vi "EventDetectionMode plane.vi"(8 "error in (no error)":errorcluster, 11 "SetupInfo_IN":T1={"ConfigParameters_Analog"={"JAI camera fps"=240.0, "Bi-Lateral Galvo xy scan range (V)"=0.7, "Bi-Lateral Galvo xy scan frequency (Hz)"=500, "AOM Blind percent (%)"=0.1, "AOM start blind percent (%) "=70.0, "ROI threshold"=1.0, "AO Sampling rate"=1000000.0}, "ConfigParameters_Digital"={"Steps per volume"=25.0, "Time per volume (s)"=0.4, "OG start layer"=15.0, "Objective Lin Rising Vel (micron/ms）"=1.0, "Image depth (micron)"=200.0, "OG latency (s)"=10.0, "OG repitation"=3.0, "OG end layer"=17.0, "Shock1 duration (s)"=0.001, "Shock2 duration (s)"=0.001, "Shock3 duration (s)"=0.01, "Shock4 duration (s)"=0.01, "Shock5 duration (s)"=0.1, "Shock duration_New"=[]}, "ConfigParameters_Other1"={"Frontal Galvo xy scan range (V)"=0.14, "Frontal Galvo xy scan frequency (Hz)"=500, "PFI 0 digital clock frequency"=500000.0, "Window size for layer index"=0.5, "sCMOS fps"=95.0}, "ConfigParameters_Others2"={"#Trials baseline"=6, "#Trials test"=6, "Time before acq. (s)"=360.0, "Time before test (s)"=600.0, "#Blocks acquisition"=5, "Inter-trial interval baseline (s)"=60.0, "#Trials per acquition block"=6, "Inter-block interval acquisition (s)"=360.0, "Inter-trial interval acquisition (s)"=20.0, "Flash latency (s)"=10.0, "Flash duration (s)"=3.2, "Response duration (s)"=10.0, "MaxTimeEventDetection (s)"=6, "StimType"=enum."Flash", "#MaxEvents"=6}, "ProcessParametersOut"={"stand Z vol Acquisition time (s)"=0.2631578947368421, "stand Z vol Backward time (s)"=0.13684210526315793, "Objective scan volt"=5.0, "Bi-lateral Galvo Z scan volt"=0.1800000180000018, "Frontal Galvo Z scan volt"=0.14940000509752818, "Objective step length (micron)"=8.0, "OG Z volet Linear Dec time (s)"=0.024, "OG Z vol Stim. steps time (s)"=0.031578947368421054, "OG Z vol Linear Acc time (s)"=0.112, "#Vol. of flash"=8, "#Vol. of shock"=1, "#Vol. bef flash"=25, "#Vol. aft flash"=17, "OG Z vol Linear Dec time (s)"=0.112, "OG Z vol time (s)"=0.39073684210526316, "Stack duration"=[0.001, 0.001, 0.01, 0.01, 0.1], "AOM stand. value size"=400000, "Plane indexing length"=0, "#Vol. blank"=0, "#Vol. blank before acq"=1000000, "#Vol. blank before test"=263158, " #Inter-block interval acquisition (Ed-St Vol)"=1000000}, "WaveformParameters"={"stand Z vol Acquisition samp info"={"Fs"=1000000.0, "#s"=263158.0}, "stand Z vol Backward samp info"={"Fs"=1000000.0, "#s"=136842.0}, "OG Z vol Linear Acc samp info"={"Fs"=1000000.0, "#s"=112000.0}, "OG Z vol Stim. steps samp info"={"Fs"=1000000.0, "#s"=31579.0}, "OG Z volet Linear Dec samp info"={"Fs"=1000000.0, "#s"=24000.0}, "OG Z vol Linear Dec samp info"={"Fs"=1000000.0, "#s"=112000.0}, "OG Z vol samp info"={"Fs"=1000000.0, "#s"=390737.0}, "stand Z vol backforth samp info"={"Fs"=1000000.0, "#s"=400000.0}}, "AnalogWaveform"={"Bi-lateral Galvo Z stand waveform"={"t0"=timestamp(0 s since 1904-01-01), "dt"=1.0, "Y"=[]}, "Frontal Galvo Z stand waveform"={"t0"=timestamp(0 s since 1904-01-01), "dt"=1.0, "Y"=[]}, "Bi-lateral Galvo XY stand waveform"={"t0"=timestamp(0 s since 1904-01-01), "dt"=1.0, "Y"=[]}, "Frontal Galvo XY stand waveform"={"t0"=timestamp(0 s since 1904-01-01), "dt"=1.0, "Y"=[]}, "sCMOS stand waveform"={"t0"=timestamp(0 s since 1904-01-01), "dt"=1.0, "Y"=[]}, "Detection objective stand waveform"={"t0"=timestamp(0 s since 1904-01-01), "dt"=1.0, "Y"=[]}, "AOM stand waveform"={"t0"=timestamp(0 s since 1904-01-01), "dt"=1.0, "Y"=[]}, "PFI 0 clock stand waveform"={"t0"=timestamp(0 s since 1904-01-01), "dt"=1.0, "Y"=[]}, "Bi-lateral Galvo Z OG waveform"={"t0"=timestamp(0 s since 1904-01-01), "dt"=1.0, "Y"=[]}, "Bi-lateral Galvo XY OG waveform"={"t0"=timestamp(0 s since 1904-01-01), "dt"=1.0, "Y"=[]}, "Frontal Galvo Z OG waveform"={"t0"=timestamp(0 s since 1904-01-01), "dt"=1.0, "Y"=[]}, "Frontal Galvo XY OG waveform"={"t0"=timestamp(0 s since 1904-01-01), "dt"=1.0, "Y"=[]}, "sCMOS OG waveform"={"t0"=timestamp(0 s since 1904-01-01), "dt"=1.0, "Y"=[]}, "Detection objective OG waveform"={"t0"=timestamp(0 s since 1904-01-01), "dt"=1.0, "Y"=[]}, "AOM OG waveform"={"t0"=timestamp(0 s since 1904-01-01), "dt"=1.0, "Y"=[]}, "PFI 0 clock OG wavee"={"t0"=timestamp(0 s since 1904-01-01), "dt"=1.0, "Y"=[]}, "sCMOS blank waveform"={"t0"=timestamp(0 s since 1904-01-01), "dt"=1.0, "Y"=[]}, "All analog OG wave"=[], "All analog stand wave"=[], "All analog blank wave"=[], "BufferWaveform_Analog"=[], "Bi-lateral Galvo Z XY"={"t0"=timestamp(0 s since 1904-01-01), "dt"=1.0, "Y"=[]}, "Frontal Galvo Z XY"={"t0"=timestamp(0 s since 1904-01-01), "dt"=1.0, "Y"=[]}, "sCMOS Trigger XY"={"t0"=timestamp(0 s since 1904-01-01), "dt"=1.0, "Y"=[]}, "Detection objective XY"={"t0"=timestamp(0 s since 1904-01-01), "dt"=1.0, "Y"=[]}, "AOM XY"={"t0"=timestamp(0 s since 1904-01-01), "dt"=1.0, "Y"=[]}, "Analog_XY"=[]}, "DigitalWaveform"={"AllDigitalStandWave"=[], "AllDigialEvokedWave"=[], "AllDigialOGWave"=[], "AllDigitalPairWave_1"=[], "AllDigitalPairWave_2"=[], "AllDigitalPairWave_3"=[], "AllDigitalPairWave_4"=[], "AllDigitalPairWave_5"=[], "Plane Indexing"={"t0"=timestamp(0 s since 1904-01-01), "dt"=0.0, "Y"={"transitions"=[], "data"=[]}, "error"={"status"=FALSE, "code"=37421928, "source"=""}}, "Plane indexing P0.5 OG"={"t0"=timestamp(0 s since 1904-01-01), "dt"=0.0, "Y"={"transitions"=[], "data"=[]}, "error"={"status"=FALSE, "code"=37421928, "source"=""}}, "AllDigitalPairWaves"=[], "BufferWaveform_Digital"=[], "AllDigitalBlankWave"=[], "Digial_XY"=[], "Digital_XY_flash"=[], "Digial_XY DMD"=[]}, "PhysicalResource"={"PhysicalChannels_AI"="", "PhysicalChannels_AO"="", "PhysicalChannels_DO"="", "Task_AnalogOutput"="", "Task_DigitalOutput"="", "Task_AnalogInput"=""}, "ControlsRef"={"Mode_1"=refnum, "EventDetectionMode"=refnum, "Mode_2A"=refnum, "StimulationMode"=refnum, "Mode_2B"=refnum, "ErrorMeg"=refnum}, "test"=""} {"ConfigParameters_Other1"."Frontal Galvo xy scan frequency (Hz)" min=500 max=500; "ConfigParameters_Other1"."Frontal Galvo xy scan range (V)" min=0.0 max=1.5; "ConfigParameters_Analog"."AOM start blind percent (%)" min=10.0 max=90.0; "ConfigParameters_Analog"."AOM Blind percent (%)" min=0.1 max=100.0; "ConfigParameters_Analog"."Bi-Lateral Galvo xy scan frequency (Hz)" min=500 max=500; "ConfigParameters_Analog"."Bi-Lateral Galvo xy scan range (V)" min=0.0 max=1.5}) -> (0 "error out":errorcluster, 3 "SetupInfo_OUT":T1={"ConfigParameters_Analog"={"JAI camera fps"=240.0, "Bi-Lateral Galvo xy scan range (V)"=0.7, "Bi-Lateral Galvo xy scan frequency (Hz)"=500, "AOM Blind percent (%)"=0.1, "AOM start blind percent (%) "=70.0, "ROI threshold"=1.0, "AO Sampling rate"=1000000.0}, "ConfigParameters_Digital"={"Steps per volume"=25.0, "Time per volume (s)"=0.4, "OG start layer"=15.0, "Objective Lin Rising Vel (micron/ms）"=1.0, "Image depth (micron)"=200.0, "OG latency (s)"=10.0, "OG repitation"=3.0, "OG end layer"=17.0, "Shock1 duration (s)"=0.001, "Shock2 duration (s)"=0.001, "Shock3 duration (s)"=0.01, "Shock4 duration (s)"=0.01, "Shock5 duration (s)"=0.1, "Shock duration_New"=[]}, "ConfigParameters_Other1"={"Frontal Galvo xy scan range (V)"=0.14, "Frontal Galvo xy scan frequency (Hz)"=500, "PFI 0 digital clock frequency"=500000.0, "Window size for layer index"=0.5, "sCMOS fps"=95.0}, "ConfigParameters_Others2"={"#Trials baseline"=6, "#Trials test"=6, "Time before acq. (s)"=360.0, "Time before test (s)"=600.0, "#Blocks acquisition"=5, "Inter-trial interval baseline (s)"=60.0, "#Trials per acquition block"=6, "Inter-block interval acquisition (s)"=360.0, "Inter-trial interval acquisition (s)"=20.0, "Flash latency (s)"=10.0, "Flash duration (s)"=3.2, "Response duration (s)"=10.0, "MaxTimeEventDetection (s)"=6, "StimType"=enum."Flash", "#MaxEvents"=6}, "ProcessParametersOut"={"stand Z vol Acquisition time (s)"=0.2631578947368421, "stand Z vol Backward time (s)"=0.13684210526315793, "Objective scan volt"=5.0, "Bi-lateral Galvo Z scan volt"=0.1800000180000018, "Frontal Galvo Z scan volt"=0.14940000509752818, "Objective step length (micron)"=8.0, "OG Z volet Linear Dec time (s)"=0.024, "OG Z vol Stim. steps time (s)"=0.031578947368421054, "OG Z vol Linear Acc time (s)"=0.112, "#Vol. of flash"=8, "#Vol. of shock"=1, "#Vol. bef flash"=25, "#Vol. aft flash"=17, "OG Z vol Linear Dec time (s)"=0.112, "OG Z vol time (s)"=0.39073684210526316, "Stack duration"=[0.001, 0.001, 0.01, 0.01, 0.1], "AOM stand. value size"=400000, "Plane indexing length"=0, "#Vol. blank"=0, "#Vol. blank before acq"=1000000, "#Vol. blank before test"=263158, " #Inter-block interval acquisition (Ed-St Vol)"=1000000}, "WaveformParameters"={"stand Z vol Acquisition samp info"={"Fs"=1000000.0, "#s"=263158.0}, "stand Z vol Backward samp info"={"Fs"=1000000.0, "#s"=136842.0}, "OG Z vol Linear Acc samp info"={"Fs"=1000000.0, "#s"=112000.0}, "OG Z vol Stim. steps samp info"={"Fs"=1000000.0, "#s"=31579.0}, "OG Z volet Linear Dec samp info"={"Fs"=1000000.0, "#s"=24000.0}, "OG Z vol Linear Dec samp info"={"Fs"=1000000.0, "#s"=112000.0}, "OG Z vol samp info"={"Fs"=1000000.0, "#s"=390737.0}, "stand Z vol backforth samp info"={"Fs"=1000000.0, "#s"=400000.0}}, "AnalogWaveform"={"Bi-lateral Galvo Z stand waveform"={"t0"=timestamp(0 s since 1904-01-01), "dt"=1.0, "Y"=[]}, "Frontal Galvo Z stand waveform"={"t0"=timestamp(0 s since 1904-01-01), "dt"=1.0, "Y"=[]}, "Bi-lateral Galvo XY stand waveform"={"t0"=timestamp(0 s since 1904-01-01), "dt"=1.0, "Y"=[]}, "Frontal Galvo XY stand waveform"={"t0"=timestamp(0 s since 1904-01-01), "dt"=1.0, "Y"=[]}, "sCMOS stand waveform"={"t0"=timestamp(0 s since 1904-01-01), "dt"=1.0, "Y"=[]}, "Detection objective stand waveform"={"t0"=timestamp(0 s since 1904-01-01), "dt"=1.0, "Y"=[]}, "AOM stand waveform"={"t0"=timestamp(0 s since 1904-01-01), "dt"=1.0, "Y"=[]}, "PFI 0 clock stand waveform"={"t0"=timestamp(0 s since 1904-01-01), "dt"=1.0, "Y"=[]}, "Bi-lateral Galvo Z OG waveform"={"t0"=timestamp(0 s since 1904-01-01), "dt"=1.0, "Y"=[]}, "Bi-lateral Galvo XY OG waveform"={"t0"=timestamp(0 s since 1904-01-01), "dt"=1.0, "Y"=[]}, "Frontal Galvo Z OG waveform"={"t0"=timestamp(0 s since 1904-01-01), "dt"=1.0, "Y"=[]}, "Frontal Galvo XY OG waveform"={"t0"=timestamp(0 s since 1904-01-01), "dt"=1.0, "Y"=[]}, "sCMOS OG waveform"={"t0"=timestamp(0 s since 1904-01-01), "dt"=1.0, "Y"=[]}, "Detection objective OG waveform"={"t0"=timestamp(0 s since 1904-01-01), "dt"=1.0, "Y"=[]}, "AOM OG waveform"={"t0"=timestamp(0 s since 1904-01-01), "dt"=1.0, "Y"=[]}, "PFI 0 clock OG wavee"={"t0"=timestamp(0 s since 1904-01-01), "dt"=1.0, "Y"=[]}, "sCMOS blank waveform"={"t0"=timestamp(0 s since 1904-01-01), "dt"=1.0, "Y"=[]}, "All analog OG wave"=[], "All analog stand wave"=[], "All analog blank wave"=[], "BufferWaveform_Analog"=[], "Bi-lateral Galvo Z XY"={"t0"=timestamp(0 s since 1904-01-01), "dt"=1.0, "Y"=[]}, "Frontal Galvo Z XY"={"t0"=timestamp(0 s since 1904-01-01), "dt"=1.0, "Y"=[]}, "sCMOS Trigger XY"={"t0"=timestamp(0 s since 1904-01-01), "dt"=1.0, "Y"=[]}, "Detection objective XY"={"t0"=timestamp(0 s since 1904-01-01), "dt"=1.0, "Y"=[]}, "AOM XY"={"t0"=timestamp(0 s since 1904-01-01), "dt"=1.0, "Y"=[]}, "Analog_XY"=[]}, "DigitalWaveform"={"AllDigitalStandWave"=[], "AllDigialEvokedWave"=[], "AllDigialOGWave"=[], "AllDigitalPairWave_1"=[], "AllDigitalPairWave_2"=[], "AllDigitalPairWave_3"=[], "AllDigitalPairWave_4"=[], "AllDigitalPairWave_5"=[], "Plane Indexing"={"t0"=timestamp(0 s since 1904-01-01), "dt"=0.0, "Y"={"transitions"=[], "data"=[]}, "error"={"status"=FALSE, "code"=37421928, "source"=""}}, "Plane indexing P0.5 OG"={"t0"=timestamp(0 s since 1904-01-01), "dt"=0.0, "Y"={"transitions"=[], "data"=[]}, "error"={"status"=FALSE, "code"=37421928, "source"=""}}, "AllDigitalPairWaves"=[], "BufferWaveform_Digital"=[], "AllDigitalBlankWave"=[], "Digial_XY"=[], "Digital_XY_flash"=[], "Digial_XY DMD"=[]}, "PhysicalResource"={"PhysicalChannels_AI"="", "PhysicalChannels_AO"="", "PhysicalChannels_DO"="", "Task_AnalogOutput"="", "Task_DigitalOutput"="", "Task_AnalogInput"=""}, "ControlsRef"={"Mode_1"=refnum, "EventDetectionMode"=refnum, "Mode_2A"=refnum, "StimulationMode"=refnum, "Mode_2B"=refnum, "ErrorMeg"=refnum}, "test"=""} {"ConfigParameters_Other1"."Frontal Galvo xy scan frequency (Hz)" min=500 max=500; "ConfigParameters_Other1"."Frontal Galvo xy scan range (V)" min=0.0 max=1.5; "ConfigParameters_Analog"."AOM start blind percent (%)" min=10.0 max=90.0; "ConfigParameters_Analog"."AOM Blind percent (%)" min=0.1 max=100.0; "ConfigParameters_Analog"."Bi-Lateral Galvo xy scan frequency (Hz)" min=500 max=500; "ConfigParameters_Analog"."Bi-Lateral Galvo xy scan range (V)" min=0.0 max=1.5})   [LabVIEW 2018]
uses:
  SetupInfo.ctl
  ConfigParameters_Analog.ctl
  ConfigParameters_Digital.ctl
  ConfigParameters_Others1.ctl
  ConfigParameters_Others2.ctl
  ProcessParametersOut.ctl
  WaveformParameters.ctl
  AnalogWaveform.ctl
  DigitalWaveform.ctl
  PhysicalResource.ctl
  ControlsRef.ctl
  <vilib>/DAQmx/write.llb/DAQmx Write (Analog DBL 1Chan 1Samp).vi
  <vilib>/Analysis/baseanly.llb/Mean (DBL).vi
  <vilib>/DAQmx/create/channels.llb/DAQmx Create Channel (AO-Voltage-Basic).vi
  <vilib>/DAQmx/miscellaneous.llb/DAQmx Fill In Error Info.vi
  Trigger_Global.vi
  <vilib>/Analysis/NI_AALBase.lvlib
panel:
  out "OG?":bool
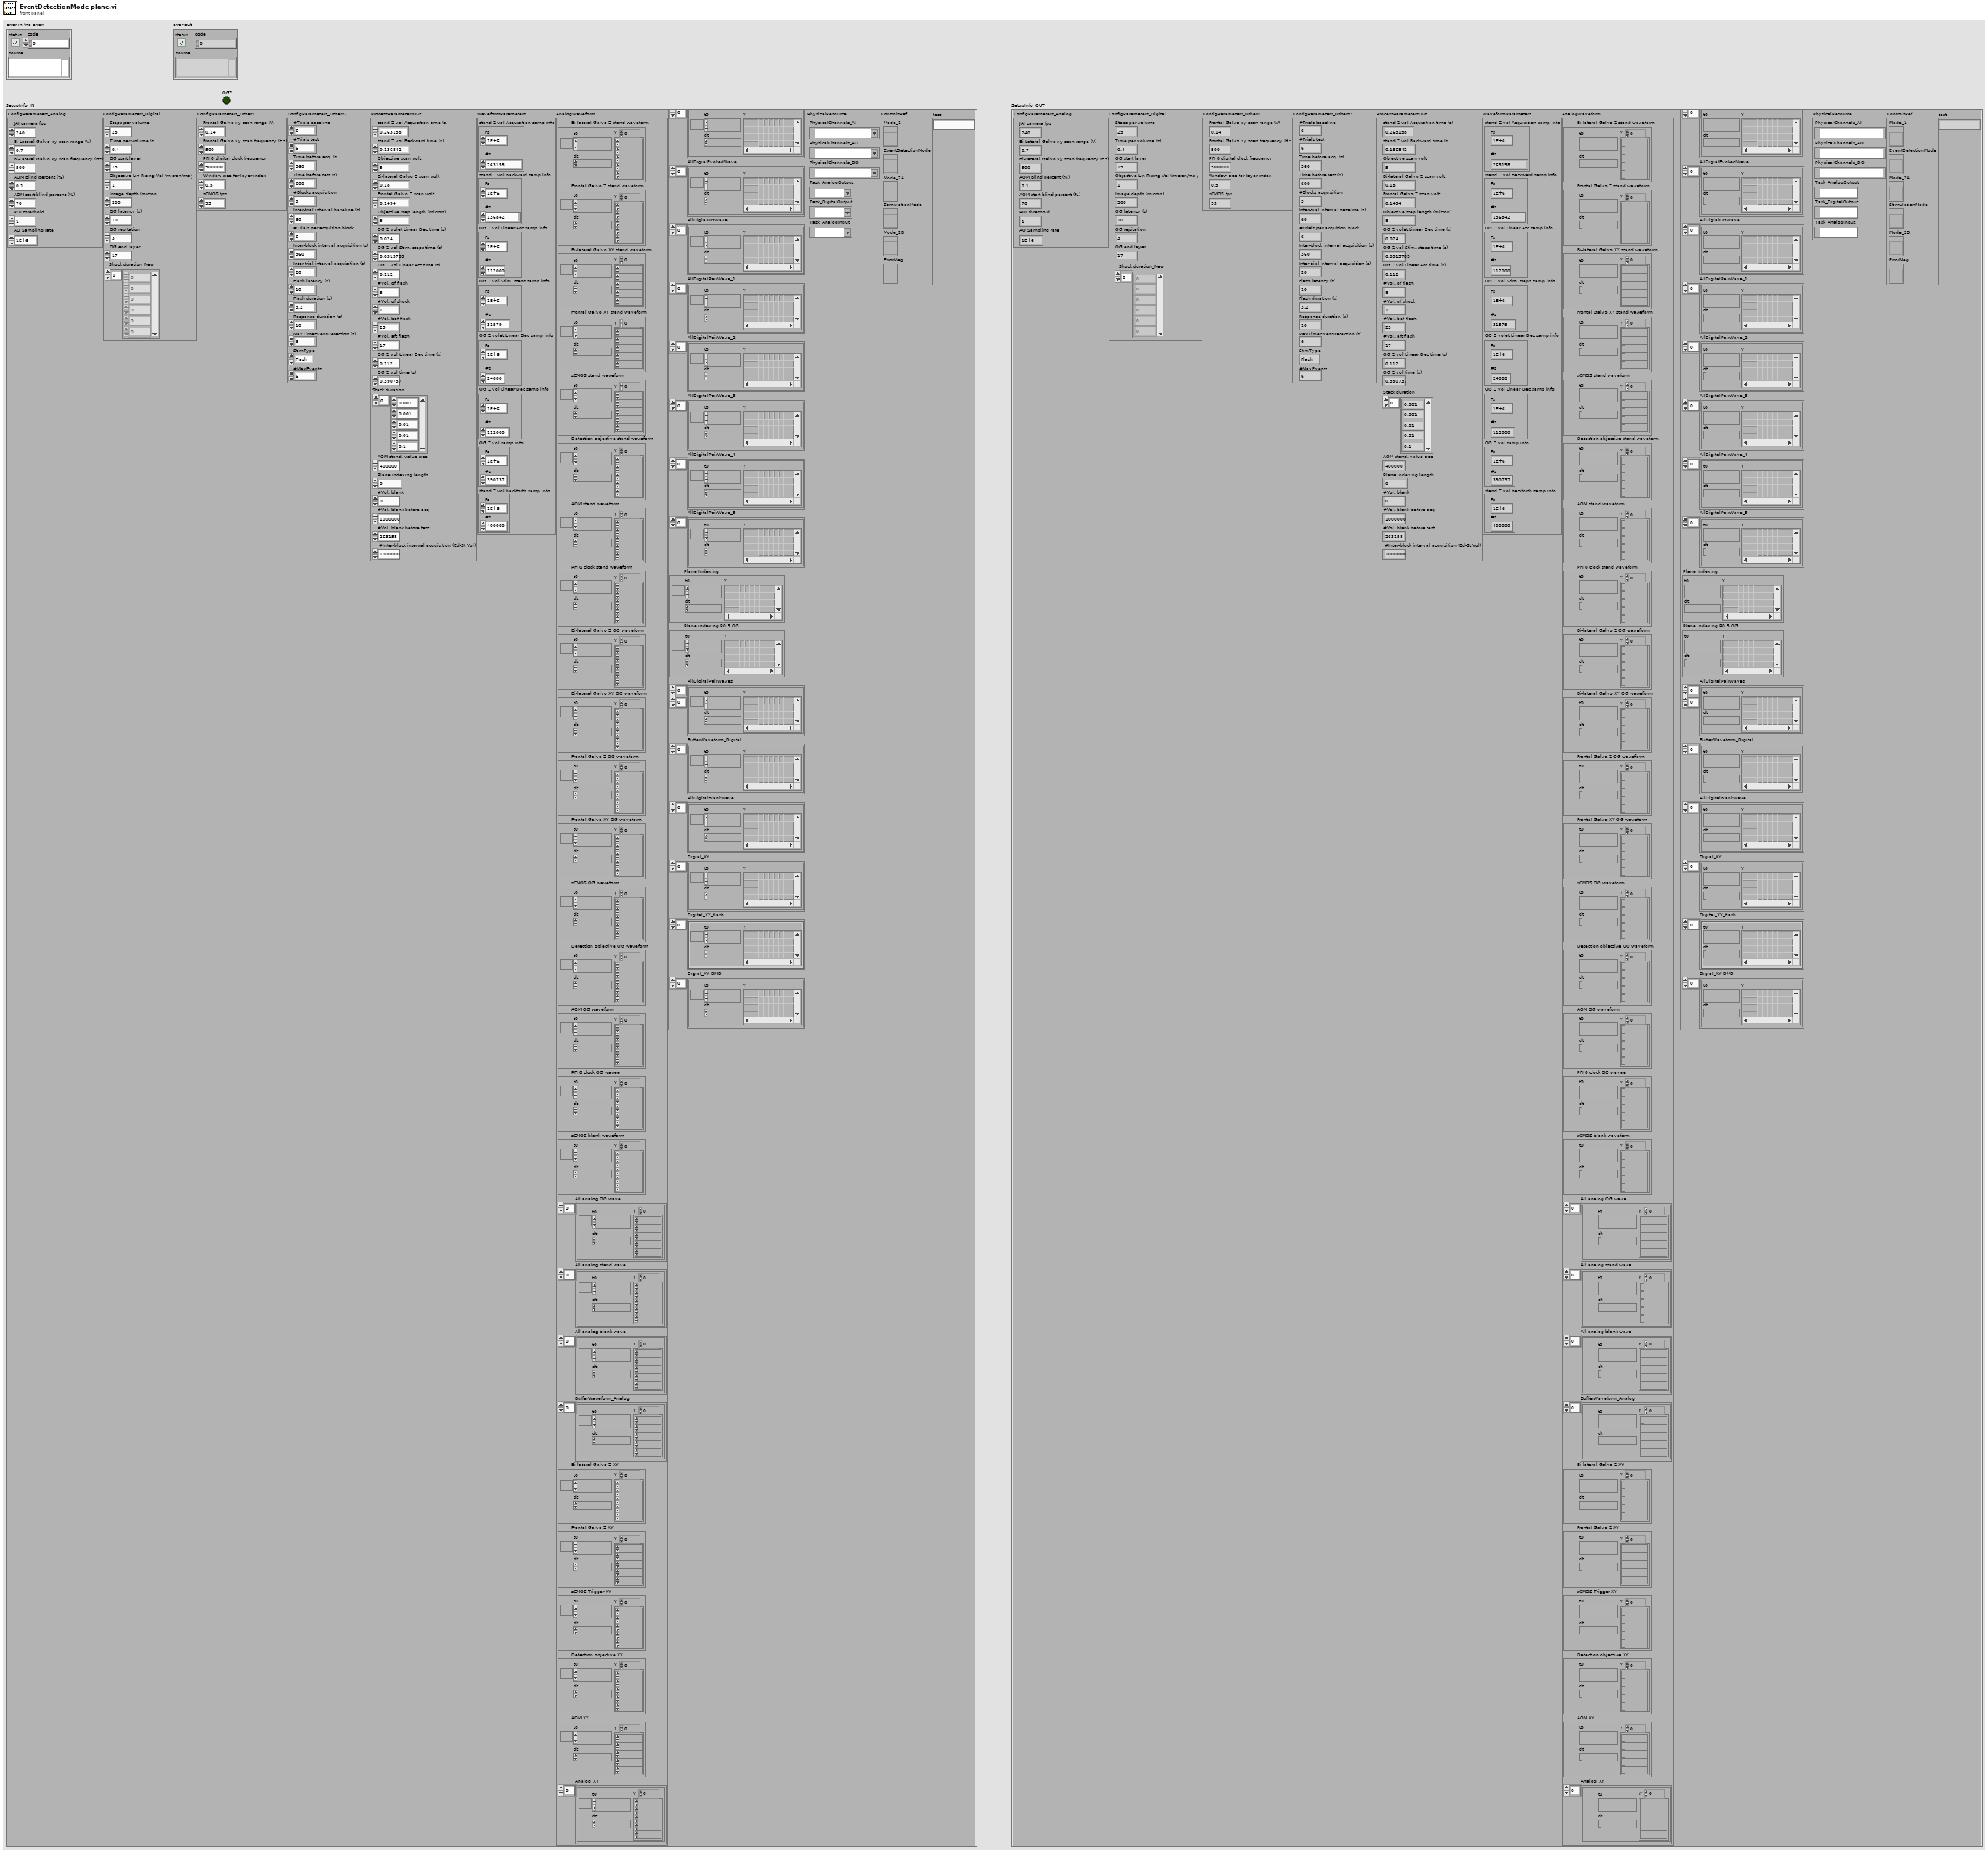
[diagram p1: front panel]
types:
  T1 = typedef "SetupInfo.ctl" = cluster{"ConfigParameters_Analog":T2, "ConfigParameters_Digital":T3, "ConfigParameters_Other1":T4, "ConfigParameters_Others2":T5, "ProcessParametersOut":T6, "WaveformParameters":T7, "AnalogWaveform":T8, "DigitalWaveform":T9, "PhysicalResource":T10, "ControlsRef":T11, "test":string}
  T2 = typedef "ConfigParameters_Analog.ctl" = cluster{"JAI camera fps":dbl, "Bi-Lateral Galvo xy scan range (V)":dbl, "Bi-Lateral Galvo xy scan frequency (Hz)":i16, "AOM Blind percent (%)":dbl, "AOM start blind percent (%) ":dbl, "ROI threshold":dbl, "AO Sampling rate":dbl}
  T3 = typedef "ConfigParameters_Digital.ctl" = cluster{"Steps per volume":dbl, "Time per volume (s)":dbl, "OG start layer":dbl, "Objective Lin Rising Vel (micron/ms）":dbl, "Image depth (micron)":dbl, "OG latency (s)":dbl, "OG repitation":dbl, "OG end layer":dbl, "Shock1 duration (s)":dbl, "Shock2 duration (s)":dbl, "Shock3 duration (s)":dbl, "Shock4 duration (s)":dbl, "Shock5 duration (s)":dbl, "Shock duration_New":dbl[]}
  T4 = typedef "ConfigParameters_Others1.ctl" = cluster{"Frontal Galvo xy scan range (V)":dbl, "Frontal Galvo xy scan frequency (Hz)":i16, "PFI 0 digital clock frequency":dbl, "Window size for layer index":dbl, "sCMOS fps":dbl}
  T5 = typedef "ConfigParameters_Others2.ctl" = cluster{"#Trials baseline":i32, "#Trials test":i32, "Time before acq. (s)":dbl, "Time before test (s)":dbl, "#Blocks acquisition":i32, "Inter-trial interval baseline (s)":dbl, "#Trials per acquition block":i32, "Inter-block interval acquisition (s)":dbl, "Inter-trial interval acquisition (s)":dbl, "Flash latency (s)":dbl, "Flash duration (s)":dbl, "Response duration (s)":dbl, "MaxTimeEventDetection (s)":i32, "StimType":enum16{"Flash", "OG"}, "#MaxEvents":i32}
  T6 = typedef "ProcessParametersOut.ctl" = cluster{"stand Z vol Acquisition time (s)":dbl, "stand Z vol Backward time (s)":dbl, "Objective scan volt":dbl, "Bi-lateral Galvo Z scan volt":dbl, "Frontal Galvo Z scan volt":dbl, "Objective step length (micron)":dbl, "OG Z volet Linear Dec time (s)":dbl, "OG Z vol Stim. steps time (s)":dbl, "OG Z vol Linear Acc time (s)":dbl, "#Vol. of flash":i32, "#Vol. of shock":i32, "#Vol. bef flash":i32, "#Vol. aft flash":i32, "OG Z vol Linear Dec time (s)":dbl, "OG Z vol time (s)":dbl, "Stack duration":dbl[], "AOM stand. value size":i32, "Plane indexing length":i32, "#Vol. blank":i32, "#Vol. blank before acq":i32, "#Vol. blank before test":i32, " #Inter-block interval acquisition (Ed-St Vol)":i32}
  T7 = typedef "WaveformParameters.ctl" = cluster{"stand Z vol Acquisition samp info":cluster{"Fs":dbl, "#s":dbl}, "stand Z vol Backward samp info":cluster{"Fs":dbl, "#s":dbl}, "OG Z vol Linear Acc samp info":cluster{"Fs":dbl, "#s":dbl}, "OG Z vol Stim. steps samp info":cluster{"Fs":dbl, "#s":dbl}, "OG Z volet Linear Dec samp info":cluster{"Fs":dbl, "#s":dbl}, "OG Z vol Linear Dec samp info":cluster{"Fs":dbl, "#s":dbl}, "OG Z vol samp info":cluster{"Fs":dbl, "#s":dbl}, "stand Z vol backforth samp info":cluster{"Fs":dbl, "#s":dbl}}
  T8 = typedef "AnalogWaveform.ctl" = cluster{"Bi-lateral Galvo Z stand waveform":waveform(dbl), "Frontal Galvo Z stand waveform":waveform(dbl), "Bi-lateral Galvo XY stand waveform":waveform(dbl), "Frontal Galvo XY stand waveform":waveform(dbl), "sCMOS stand waveform":waveform(dbl), "Detection objective stand waveform":waveform(dbl), "AOM stand waveform":waveform(dbl), "PFI 0 clock stand waveform":waveform(dbl), "Bi-lateral Galvo Z OG waveform":waveform(dbl), "Bi-lateral Galvo XY OG waveform":waveform(dbl), "Frontal Galvo Z OG waveform":waveform(dbl), "Frontal Galvo XY OG waveform":waveform(dbl), "sCMOS OG waveform":waveform(dbl), "Detection objective OG waveform":waveform(dbl), "AOM OG waveform":waveform(dbl), "PFI 0 clock OG wavee":waveform(dbl), "sCMOS blank waveform":waveform(dbl), "All analog OG wave":waveform(dbl)[], "All analog stand wave":waveform(dbl)[], "All analog blank wave":waveform(dbl)[], "BufferWaveform_Analog":waveform(dbl)[], "Bi-lateral Galvo Z XY":waveform(dbl), "Frontal Galvo Z XY":waveform(dbl), "sCMOS Trigger XY":waveform(dbl), "Detection objective XY":waveform(dbl), "AOM XY":waveform(dbl), "Analog_XY":waveform(dbl)[]}
  T9 = typedef "DigitalWaveform.ctl" = cluster{"AllDigitalStandWave":digitalwaveform[], "AllDigialEvokedWave":digitalwaveform[], "AllDigialOGWave":digitalwaveform[], "AllDigitalPairWave_1":digitalwaveform[], "AllDigitalPairWave_2":digitalwaveform[], "AllDigitalPairWave_3":digitalwaveform[], "AllDigitalPairWave_4":digitalwaveform[], "AllDigitalPairWave_5":digitalwaveform[], "Plane Indexing":digitalwaveform, "Plane indexing P0.5 OG":digitalwaveform, "AllDigitalPairWaves":digitalwaveform[][], "BufferWaveform_Digital":digitalwaveform[], "AllDigitalBlankWave":digitalwaveform[], "Digial_XY":digitalwaveform[], "Digital_XY_flash":digitalwaveform[], "Digial_XY DMD":digitalwaveform[]}
  T10 = typedef "PhysicalResource.ctl" = cluster{"PhysicalChannels_AI":tag, "PhysicalChannels_AO":tag, "PhysicalChannels_DO":tag, "Task_AnalogOutput":refnum<k21>, "Task_DigitalOutput":refnum<k21>, "Task_AnalogInput":refnum<k21>}
  T11 = typedef "ControlsRef.ctl" = cluster{"Mode_1":refnum<vi>, "EventDetectionMode":refnum<vi>, "Mode_2A":refnum<vi>, "StimulationMode":refnum<vi>, "Mode_2B":refnum<vi>, "ErrorMeg":refnum<vi>}
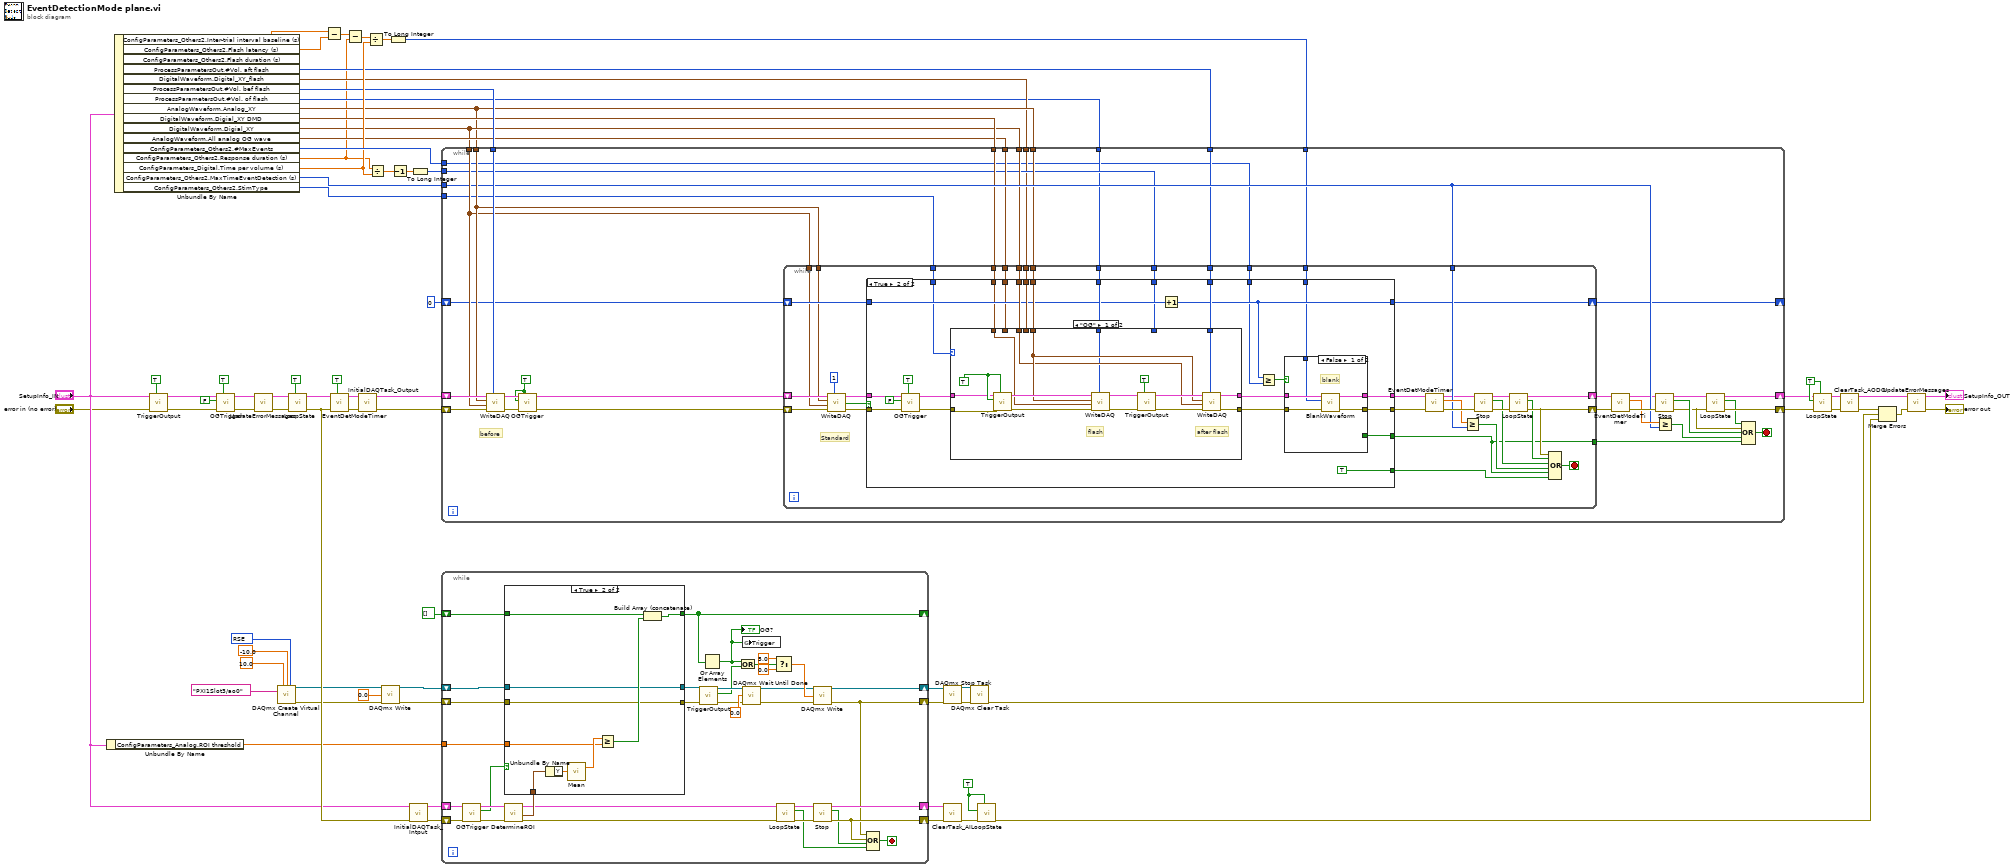
[diagram p0: block diagram]
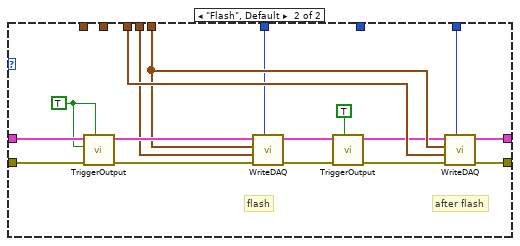
[diagram p3: hidden frame]
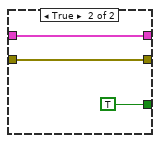
[diagram p4: hidden frame]
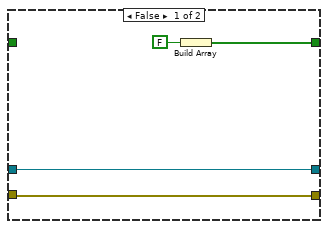
[diagram p5: hidden frame]
diagram:
  w15 = 10083 items=["Default"=-1, "RSE"=10083, "Differential"=10106, "Pseudodifferential"=12529] ("output terminal configuration")
  w57 = TRUE ("Write?")
  w64 = TRUE ("Write?")
  n1 = Unbundle By Name("SetupInfo_IN") -> ("ConfigParameters_Analog.ROI threshold"=w30:dbl)
  n2 = Unbundle By Name("SetupInfo_IN") -> ("ConfigParameters_Others2.Inter-trial interval baseline (s)"=w45:dbl, "ConfigParameters_Others2.Flash latency (s)"=w44:dbl, "ProcessParametersOut.#Vol. aft flash"=w22:i32, "DigitalWaveform.Digital_XY_flash"=w24:digitalwaveform[], "ProcessParametersOut.#Vol. bef flash"=w39:i32, "ProcessParametersOut.#Vol. of flash"=w23:i32, "AnalogWaveform.Analog_XY"=w25:waveform(dbl)[], "DigitalWaveform.Digial_XY DMD"=w28:digitalwaveform[], "DigitalWaveform.Digial_XY"=w26:digitalwaveform[], "AnalogWaveform.All analog OG wave"=w27:waveform(dbl)[], "ConfigParameters_Others2.#MaxEvents"=w63:i32, "ConfigParameters_Others2.Response duration (s)"=w1:dbl, "ConfigParameters_Digital.Time per volume (s)"=w41:dbl, "ConfigParameters_Others2.MaxTimeEventDetection (s)"=w59:i32, "ConfigParameters_Others2.StimType"=w49:enum16{"Flash", "OG"})  [unwired: 1 out]
  n3 = call "TriggerOutput.vi"("Write?"=TRUE, "error in (no error)"="error in (no error)") -> ("error out"=w10:errorcluster)  [unwired: 8 in, 1 out]
  n4 = call "OGTrigger.vi"("Write?"=TRUE, "error in (no error)"=w10, "StateIn"=FALSE) -> ("error out"=w34:errorcluster)  [unwired: 7 in, 1 out]
  n5 = call "UpdateErrorMessages.vi"("error in (no error)"=w34, "SetupInfo_IN"="SetupInfo_IN") -> ("error out"=w50:errorcluster, "SetupInfo_OUT"=w51:T1)  [unwired: 8 in]
  n6 = call-poly <vilib>:"DAQmx Create Virtual Channel.vi"("maximum value"=10.0, "minimum value"=-10.0, "output terminal configuration"=w15, "physical channels"=tag "PXI1Slot3/ao0") -> ("task out"=w6:refnum<k21>, "error out"=w5:errorcluster)  [unwired: 10 in]
  n7 = call "LoopState.vi"("Write?"=TRUE, "error in (no error)"=w50) -> ("error out"=w36:errorcluster)  [unwired: 8 in, 1 out]
  n8 = Subtract(x=w45, y=w44) -> (x-y=w43:dbl)
  n9 = call "EventDetModeTimer.vi"("Initial"=TRUE, "error in (no error)"=w36) -> ("error out"=w37:errorcluster)  [unwired: 8 in, 1 out]
  n10 = Subtract(x=w43, y=w1) -> (x-y=w42:dbl)
  n11 = call "InitialDAQTask_Output.vi"("error in (no error)"=w37, "SetupInfo_IN"=w51) -> ("error out"=w35:errorcluster, "SetupInfo_OUT"=w38:T1)  [unwired: 8 in]
  n12 = Divide(x=w42, y=w41) -> (x/y=w40:dbl)
  n13 = Divide(x=w1, y=w41) -> (x/y=w62:dbl)
  n14 = call-poly <vilib>:"DAQmx Write.vi"("task/channels in"=w6, "data"=0.0, "error in"=w5) -> ("task out"=w3:refnum<k21>, "error out"=w4:errorcluster)  [unwired: 10 in, 1 out]
  n15 = To Long Integer(number=w40) -> (32bit integer=w21:i32)
  n16 = Decrement(x=w62) -> (x-1=w61:dbl)
  n17 = call "InitialDAQTask_Intput.vi"("error in (no error)"=w36, "SetupInfo_IN"="SetupInfo_IN") -> ("error out"=w70:errorcluster, "SetupInfo_OUT"=w58:T1)  [unwired: 8 in]
  n18 = To Long Integer(number=w61) -> (32bit integer=w48:i32)
  n19 = while {
    shift-right: [w98] -> w46
    shift-left: w35 -> [w95]
    shift-right: [w73] -> w47
    shift-left: w38 -> [w96]
    tunnel: w63 -> [w77]
    tunnel: w48 -> [w81]
    tunnel: w59 -> [w90]
    tunnel: w49 -> [w82]
    tunnel: w39 -> [w94]
    tunnel: w25 -> [w92]
    tunnel: w26 -> [w91]
    tunnel: w28 -> [w86]
    tunnel: w27 -> [w85]
    tunnel: w26 -> [w84]
    tunnel: w25 -> [w83]
    tunnel: w24 -> [w80]
    tunnel: w23 -> [w79]
    tunnel: w22 -> [w78]
    tunnel: w21 -> [w76]
    shift-right: [w75] -> _
    shift-left: 0 -> [w74]
    stop <- w102 stop-if-true
    w89 = TRUE ("Write?")
    # "before"
    n20 = call "WriteDAQ.vi"("Cycle"=w94, "error in (no error)"=w95, "DigitalWaveform_In"=w91, "AnalogWaveform_In"=w92, "SetupInfo_IN"=w96) -> ("error out"=w87:errorcluster, "SetupInfo_OUT"=w93:T1)  [unwired: 4 in, 1 out]
    n21 = call "OGTrigger.vi"("Write?"=w89, "error in (no error)"=w87, "StateIn"=w89) -> ("error out"=w88:errorcluster)  [unwired: 7 in, 1 out]
    n22 = while {
      shift-right: [w119] -> w73
      shift-left: w93 -> [w112]
      shift-right: [w133] -> w71
      shift-left: w88 -> [w111]
      tunnel: w92 -> [w109]
      tunnel: w91 -> [w108]
      tunnel: w90 -> [w134]
      tunnel: w86 -> [w129]
      tunnel: w85 -> [w128]
      tunnel: w84 -> [w127]
      tunnel: w83 -> [w126]
      tunnel: w82 -> [w125]
      tunnel: w81 -> [w124]
      tunnel: w80 -> [w123]
      tunnel: w79 -> [w122]
      tunnel: w78 -> [w121]
      shift-right: [w117] -> w75
      shift-left: w74 -> [w118]
      tunnel: w77 -> [w116]
      tunnel: w76 -> [w115]
      tunnel: [w114] -> w72
      stop <- w138 stop-if-true
      # "Standard"
      n23 = call "WriteDAQ.vi"("Cycle"=1, "error in (no error)"=w111, "DigitalWaveform_In"=w108, "AnalogWaveform_In"=w109, "SetupInfo_IN"=w112) -> ("error out"=w106:errorcluster, "Trigger"=w105:bool, "SetupInfo_OUT"=w110:T1)  [unwired: 4 in]
      n24 = case shown="True" w105 {
        tunnel: w129 -> [_ w144]
        tunnel: w128 -> [_ w145]
        tunnel: w110 -> [w140 w166]
        tunnel: w127 -> [_ w165]
        tunnel: w126 -> [_ w164]
        tunnel: w125 -> [_ w146]
        tunnel: w124 -> [_ w143]
        tunnel: w123 -> [_ w163]
        tunnel: w122 -> [_ w162]
        tunnel: w121 -> [_ w161]
        tunnel: [w141 w155] -> w120
        tunnel: w106 -> [w141 w147]
        tunnel: [w140 w156] -> w119
        tunnel: w118 -> [w139 w160]
        tunnel: [w139 w159] -> w117
        tunnel: w116 -> [_ w158]
        tunnel: w115 -> [_ w153]
        tunnel: [_ w152] -> w114
        tunnel: [_ TRUE] -> w113
        frame False {
        }
        frame True {
          n25 = call "OGTrigger.vi"("Write?"=TRUE, "error in (no error)"=w147, "StateIn"=FALSE) -> ("error out"=w142:errorcluster)  [unwired: 7 in, 1 out]
          n26 = case shown="\"OG\"" w146 {
            tunnel: w166 -> [w172 w196]
            tunnel: w165 -> [w169 w195]
            tunnel: w164 -> [w170 w194]
            tunnel: w163 -> [_ w193]
            tunnel: w162 -> [w167 w192]
            tunnel: w161 -> [w171 w191]
            tunnel: [w173 w190] -> w157
            tunnel: [w174 w188] -> w148
            tunnel: w142 -> [w175 w183]
            tunnel: w145 -> [_ _]
            tunnel: w144 -> [w168 _]
            tunnel: w143 -> [_ _]
            frame "OG" {
              w177 = TRUE ("Write?")
              # "after flash"
              # "flash"
              n27 = call "TriggerOutput.vi"("Write?"=w177, "error in (no error)"=w175, "StateIn"=w177) -> ("error out"=w176:errorcluster)  [unwired: 7 in, 1 out]
              n28 = call "WriteDAQ.vi"("Cycle"=w167, "error in (no error)"=w176, "DigitalWaveform_In"=w168, "AnalogWaveform_In"=w170, "SetupInfo_IN"=w172) -> ("error out"=w178:errorcluster, "SetupInfo_OUT"=w181:T1)  [unwired: 4 in, 1 out]
              n29 = call "TriggerOutput.vi"("Write?"=TRUE, "error in (no error)"=w178) -> ("error out"=w179:errorcluster)  [unwired: 8 in, 1 out]
              n30 = call "WriteDAQ.vi"("Cycle"=w171, "error in (no error)"=w179, "DigitalWaveform_In"=w169, "AnalogWaveform_In"=w170, "SetupInfo_IN"=w181) -> ("error out"=w174:errorcluster, "SetupInfo_OUT"=w173:T1)  [unwired: 4 in, 1 out]
            }
            frame "Flash", Default {
              w184 = TRUE ("Write?")
              # "after flash"
              # "flash"
              n31 = call "TriggerOutput.vi"("Write?"=w184, "error in (no error)"=w183, "StateIn"=w184) -> ("error out"=w182:errorcluster)  [unwired: 7 in, 1 out]
              n32 = call "WriteDAQ.vi"("Cycle"=w192, "error in (no error)"=w182, "DigitalWaveform_In"=w193, "AnalogWaveform_In"=w194, "SetupInfo_IN"=w196) -> ("error out"=w185:errorcluster, "SetupInfo_OUT"=w189:T1)  [unwired: 4 in, 1 out]
              n33 = call "TriggerOutput.vi"("Write?"=TRUE, "error in (no error)"=w185) -> ("error out"=w186:errorcluster)  [unwired: 8 in, 1 out]
              n34 = call "WriteDAQ.vi"("Cycle"=w191, "error in (no error)"=w186, "DigitalWaveform_In"=w195, "AnalogWaveform_In"=w194, "SetupInfo_IN"=w189) -> ("error out"=w188:errorcluster, "SetupInfo_OUT"=w190:T1)  [unwired: 4 in, 1 out]
            }
          }
          n35 = Increment(x=w160) -> (x+1=w159:i32)
          n36 = Greater Or Equal?(x=w159, y=w158) -> (x >= y?=w154:bool)
          n37 = case shown="False" w154 {
            tunnel: w148 -> [w201 w203]
            tunnel: w157 -> [w200 w204]
            tunnel: [w199 w204] -> w156
            tunnel: [w198 w203] -> w155
            tunnel: w153 -> [w197 _]
            tunnel: [_ TRUE] -> w152
            frame False {
              # "blank"
              n38 = call "BlankWaveform.vi"("error in (no error)"=w201, "Cycle"=w197, "SetupInfo_IN"=w200) -> ("error out"=w198:errorcluster, "SetupInfo_OUT"=w199:T1)  [unwired: 7 in]
            }
            frame True {
            }
          }
        }
      }
      n39 = call "EventDetModeTimer.vi"("error in (no error)"=w120) -> ("error out"=w136:errorcluster, "TimerOut(s)"=w135:dbl)  [unwired: 9 in]
      n40 = Greater Or Equal?(x=w135, y=w134) -> (x >= y?=w130:bool)
      n41 = call "Stop.vi"("error in (no error)"=w136) -> ("error out"=w137:errorcluster, "StateOut"=w131:bool)  [unwired: 9 in]
      n42 = call "LoopState.vi"("error in (no error)"=w137) -> ("error out"=w133:errorcluster, "StateOut"=w132:bool)  [unwired: 9 in]
      n43 = Compound Arithmetic op=OR(w133, w132, w131, w130, w114, w113) -> (w138:bool)
    }
    n44 = call "EventDetModeTimer.vi"("error in (no error)"=w71) -> ("error out"=w103:errorcluster, "TimerOut(s)"=w101:dbl)  [unwired: 9 in]
    n45 = call "Stop.vi"("error in (no error)"=w103) -> ("error out"=w99:errorcluster, "StateOut"=w104:bool)  [unwired: 9 in]
    n46 = Greater Or Equal?(x=w101, y=w90) -> (x >= y?=w100:bool)
    n47 = call "LoopState.vi"("error in (no error)"=w99) -> ("error out"=w98:errorcluster, "StateOut"=w97:bool)  [unwired: 9 in]
    n48 = Compound Arithmetic op=OR(w97, w99, w104, w100, w72) -> (w102:bool)
  }
  n49 = while {
    shift-right: [w235] -> w69
    shift-left: w70 -> [w227]
    shift-right: [w229] -> w68
    shift-left: w58 -> [w225]
    shift-right: [w222] -> _
    shift-left: bool[] [] -> [w224]
    tunnel: w30 -> [w223]
    shift-right: [w217] -> w12
    shift-left: w3 -> [w220]
    shift-right: [w209] -> w13
    shift-left: w4 -> [w218]
    stop <- w233 stop-if-true
    n50 = call "OGTrigger.vi"("error in (no error)"=w227) -> ("error out"=w228:errorcluster, "StateOut"=w221:bool)  [unwired: 9 in]
    n51 = call "DetermineROI.vi"("error in (no error)"=w228, "SetupInfo_IN"=w225) -> ("error out"=w226:errorcluster, "data"=w230:waveform(dbl), "SetupInfo_OUT"=w229:T1)  [unwired: 7 in]
    n52 = case shown="True" w221 {
      tunnel: w230 -> [_ w242]
      tunnel: [w238 w243] -> w222
      tunnel: w224 -> [_ w246]
      tunnel: w223 -> [_ w244]
      tunnel: w220 -> [w237 w241]
      tunnel: [w237 w241] -> w219
      tunnel: [w236 w240] -> w216
      tunnel: w218 -> [w236 w240]
      frame False {
        n53 = Build Array(FALSE) -> (w238:bool[])
      }
      frame True {
        n54 = Unbundle By Name(w242) -> ("Y"=w247:dbl[])
        n55 = call-poly <vilib>:"Mean.vi"("X"=w247) -> ("mean"=w248:dbl)  [unwired: 1 out]
        n56 = Greater Or Equal?(x=w248, y=w244) -> (x >= y?=w245:bool)
        n57 = Build Array (concatenate)(w246, w245) -> (w243:bool[])
      }
    }
    n58 = call "TriggerOutput.vi"("error in (no error)"=w216) -> ("error out"=w206:errorcluster, "StateOut"=w215:bool)  [unwired: 9 in]
    n59 = Or Array Elements(Boolean array=w222) -> (logical OR=w214:bool)
    "OG?" <- w214
    n60 = Compound Arithmetic op=OR(w214, w215) -> (w213:bool)
    n61 = global write "Trigger_Global.vi" "Trigger"(w214) -> ()
    n62 = call <vilib>:"DAQmx Wait Until Done.vi"("task/channels in"=w219, "timeout (sec)"=0.0, "error in"=w206) -> ("task out"=w208:refnum<k21>, "error out"=w205:errorcluster)  [unwired: 11 in]
    n63 = Select(t=5.0, s=w213, f=0.0 ("data")) -> (s? t:f=w210:dbl)
    n64 = call "LoopState.vi"("error in (no error)"=w226) -> ("error out"=w232:errorcluster, "StateOut"=w231:bool)  [unwired: 9 in]
    n65 = call-poly <vilib>:"DAQmx Write.vi"("task/channels in"=w208, "data"=w210, "error in"=w205) -> ("task out"=w217:refnum<k21>, "error out"=w209:errorcluster)  [unwired: 10 in, 1 out]
    n66 = call "Stop.vi"("error in (no error)"=w232) -> ("error out"=w235:errorcluster, "StateOut"=w234:bool)  [unwired: 9 in]
    n67 = Compound Arithmetic op=OR(w209, w235, w234, w231) -> (w233:bool)
  }
  n68 = call <vilib>:"DAQmx Stop Task.vi"("task/channels in"=w12, "error in"=w13) -> ("task out"=w19:refnum<k21>, "error out"=w18:errorcluster)  [unwired: 12 in]
  n69 = call "ClearTask_AI.vi"("error in (no error)"=w69, "SetupInfo_IN"=w68) -> ("error out"=w56:errorcluster)  [unwired: 8 in, 1 out]
  n70 = call <vilib>:"DAQmx Clear Task.vi"("task in"=w19, "error in"=w18) -> ("error out"=w7:errorcluster)  [unwired: 13 in]
  n71 = call "LoopState.vi"("Write?"=w57, "error in (no error)"=w56, "StateIn"=w57) -> ("error out"=w8:errorcluster)  [unwired: 7 in, 1 out]
  n72 = call "LoopState.vi"("Write?"=w64, "error in (no error)"=w46, "StateIn"=w64) -> ("error out"=w65:errorcluster)  [unwired: 7 in, 1 out]
  n73 = call "ClearTask_AODO.vi"("error in (no error)"=w65, "SetupInfo_IN"=w47) -> ("error out"=w67:errorcluster, "SetupInfo_OUT"=w54:T1)  [unwired: 8 in]
  n74 = Merge Errors(w67, w7, w8) -> (w55:errorcluster)
  n75 = call "UpdateErrorMessages.vi"("error in (no error)"=w55, "SetupInfo_IN"=w54) -> ("error out"=→"error out":errorcluster, "SetupInfo_OUT"=→"SetupInfo_OUT":T1)  [unwired: 8 in]
